vi "GetOutputWireBranches.vi"(6 "error in":errorcluster, 9 "Structure in":refnum<class "Structure.lvclass">) -> (0 "error out":errorcluster, 3 "Structure out":refnum<class "Structure.lvclass">, 4 "branches":string[](array[string]))   [LabVIEW 2014, in "Structure.lvclass"]
uses:
  Structure.lvclass
  Tunnel/Tunnel.lvclass
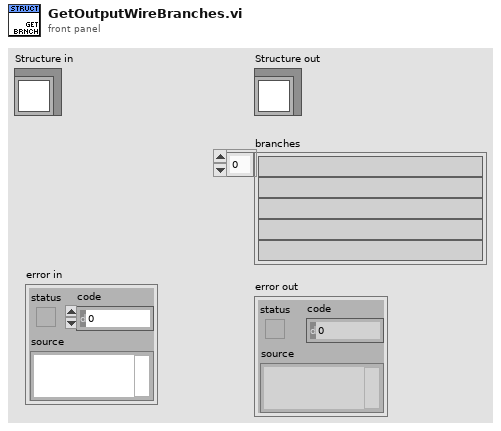
[diagram p1: front panel]
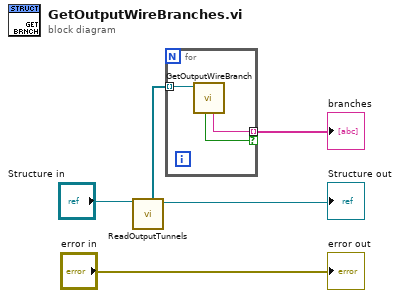
[diagram p0: block diagram]
diagram:
  n1 = call-dynamic "ReadOutputTunnels.vi"("Structure in"="Structure in") -> ("Structure out"=→"Structure out":refnum<class "Structure.lvclass">, "outputs"=w3:refnum<class "Tunnel.lvclass">[])  [unwired: 7 in]
  n2 = for {
    tunnel: w3 -> [w8] mode=indexing
    tunnel: [w7] -> w2 mode=indexing if=w6
    n3 = call-dynamic "GetOutputWireBranch.vi"("Tunnel in"=w8) -> ("branches"=w7:string, "branched"=w6:bool)  [unwired: 5 in, 2 out]
  }
  "branches" <- w2
  "error out" <- "error in"
